vi "Heater.vi"(0 "Heater in":refnum<class "Heater_v2.lvclass">, 1 "Z_ASetState":T4, 2 "ALRs":bool[](array[boolean])=[FALSE, FALSE, FALSE], 5 "ZY_control":T3 {"Y_H" step=1.0; "SP" step=0.01 format="%.2f"}, 7 "PV":dbl step=0.01 format="%.2f", 9 "PV state":T2, 11 "error in (no error)":errorcluster, 12 "ALR_Status":T1[](array[typedef]), 13 "DI":bool[](array[boolean])) -> (4 "Heater out":refnum<class "Heater_v2.lvclass">, 6 "ZY_State":T6 {"Y"."Y_Set" format="%.2f"; "Y"."SP" step=0.01 format="%.2f"; "Y"."Y" format="%.2f"; "Y"."PV" step=0.01 format="%.2f"; "Y"."SP_Set" step=0.01 format="%.2f"}, 8 "Y":dbl format="%.2f", 10 "YB":bool[](array[boolean]), 14 "ALR_ON":bool[](array[boolean]), 15 "error out":errorcluster)   [LabVIEW 2019, in "Heater_v2.lvclass"]
uses:
  Heater_v2.lvclass
  ctl/Z_State.ctl
  Heating.lvlib
  Alarms/Ctl/ALR_Status_short.ctl
  Alarms/Alarms.lvlib
  Inputs/Ctl/Parameter State short.ctl
  Inputs/Inputs.lvlib
  ctl/Y_state.ctl
  ctl/Y_source.ctl
  ctl/Y_short.ctl
  ctl/ZM_State.ctl
  ctl/Z_source.ctl
  ctl/Z.ctl
  ctl/ZY_state_short.ctl
  REG/HE_reg.lvclass
  HE_state_v2/HE_state_v2.lvclass
  C:/my_projects/projects/Algorithms/Labview/19/Heating/heating1/HE_state_v2/HE_state_v2.lvclass
  C:/my_projects/projects/Algorithms/Labview/19/Heating/heating1/Z_state_v2/HE_Z_state_v2.lvclass
  C:/my_projects/projects/Algorithms/Labview/19/Heating/heating1/ZM_state/HE_ZM_state.lvclass
  C:/my_projects/projects/Algorithms/Labview/19/Sequence/State/State.lvclass
  ctl/ZY_control.ctl
panel:
  # "0 bit - Alarm level 1\n1 bit - Alarm level 2\n2 bit - Alarm level 3"
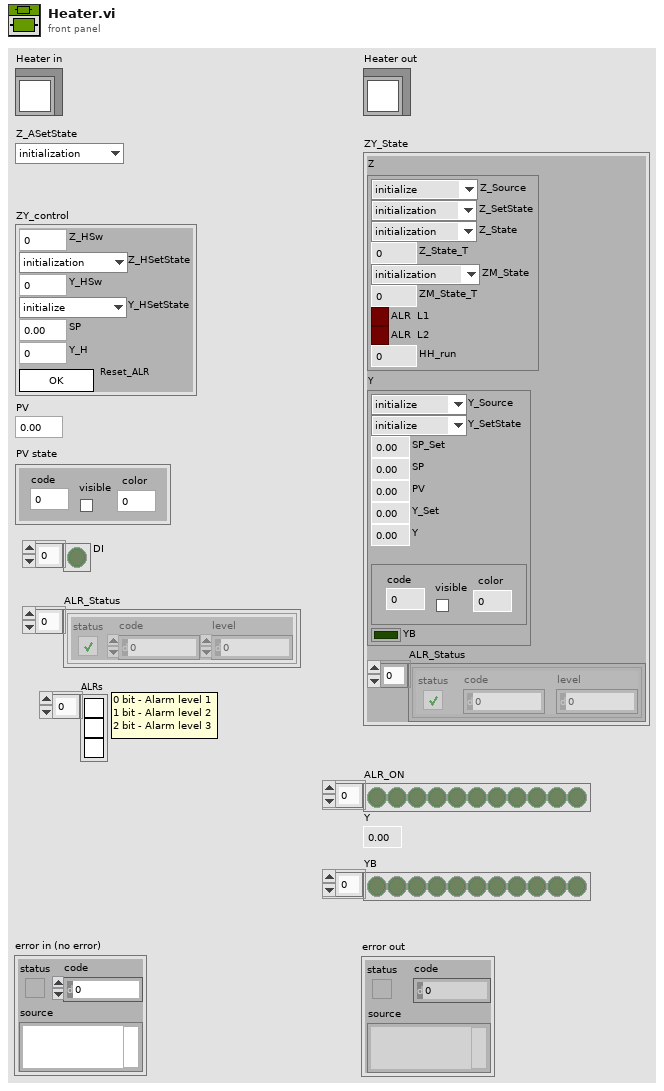
[diagram p1: front panel]
types:
  T1 = typedef "Alarms.lvlib/ALR_Status_short.ctl" = cluster{"status":bool, "code":i32, "level":i32}
  T2 = typedef "Inputs.lvlib/Parameter State short.ctl" = cluster{"code":i32, "visible":bool, "color":u32}
  T3 = typedef "Heating.lvlib/ZY_control.ctl" = cluster{"Z_HSw":u8, "Z_HSetState":T4, "Y_HSw":u8, "Y_HSetState":T5, "SP":dbl, "Y_H":dbl, "Reset_ALR":bool}
  T4 = typedef "Heating.lvlib/Z_State.ctl" = enum8{"initialization", "alarm", "disabled", "not ready", "stop ready", "reserv", "switched off", "reserv2", "switched on", "check", "on min", "decrease out", "on", "increase out", "on max"}
  T5 = typedef "Heating.lvlib/Y_state.ctl" = enum8{"initialize", "alarm", "min", "stop", "hand", "auto", "max"}
  T6 = typedef "Heating.lvlib/ZY_state_short.ctl" = cluster{"Z":T7, "Y":T10, "ALR_Status":T1[]}
  T7 = typedef "Heating.lvlib/Z.ctl" = cluster{"Z_Source":T8, "Z_SetState":T4, "Z_State":T4, "Z_State_T":u32, "ZM_State":T9, "ZM_State_T":u32, "ALR  L1":bool, "ALR  L2":bool, "HH_run":u64}
  T8 = typedef "Heating.lvlib/Z_source.ctl" = enum8{"initialize", "local disabled", "local hand", "hand", "auto", "dist"}
  T9 = typedef "Heating.lvlib/ZM_State.ctl" = enum8{"initialization", "stop", "start_cmd", "contactor_on_cmd", "heating", "on", "stop_cmd", "power_down", "contactor_off_cmd", "cooling", "restart_delay"}
  T10 = typedef "Heating.lvlib/Y_short.ctl" = cluster{"Y_Source":T11, "Y_SetState":T5, "SP_Set":dbl, "SP":dbl, "PV":dbl, "Y_Set":dbl, "Y":dbl, "Y_State":T2, "YB":bool}
  T11 = typedef "Heating.lvlib/Y_source.ctl" = enum8{"initialize", "local disabled", "local hand", "hand", "auto", "dist"}
  T12 = typedef "Heating.lvlib/Z_control.ctl" = cluster{"Z_HSw":u8, "Z_HSetState":T4, "Z_ASetState":T4, "Z_DSetState":T4}
  T13 = typedef "Heating.lvlib/Y_control.ctl" = cluster{"Y_HSw":u8, "Y_HSetState":T5, "Y_ASetState":T5, "Y_DSetState":T5}
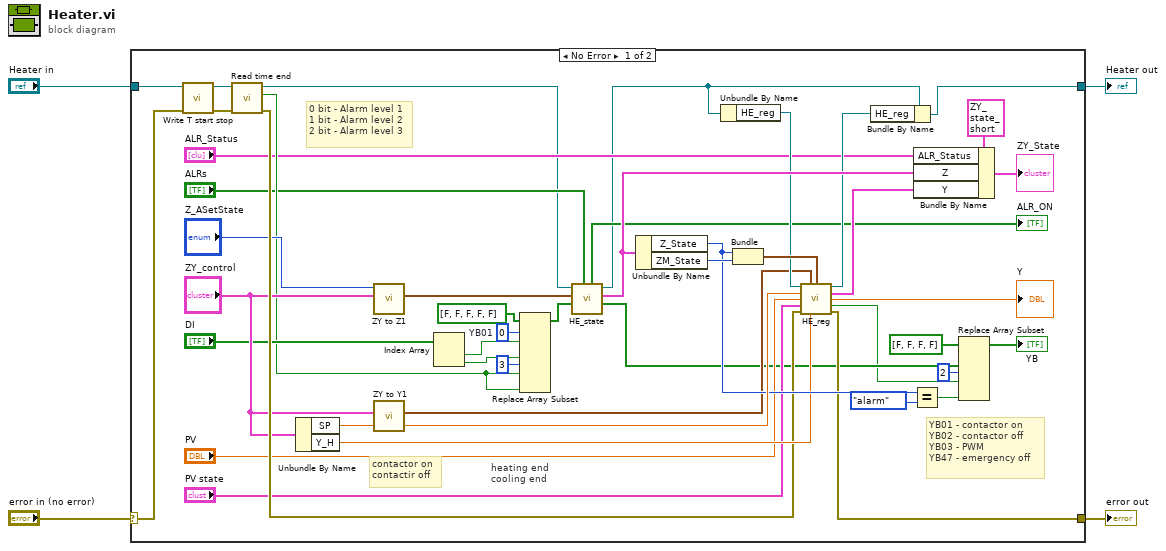
[diagram p0: block diagram]
diagram:
  n1 = case shown="No Error" "error in (no error)" {
    selector: "error in (no error)" -> [w29 w51]
    tunnel: [w27 w51] -> w3
    tunnel: [w30 w50] -> w1
    tunnel: "Heater in" -> [w25 w50]
    frame No Error {
      w49 = 0  # YB01
      # "0 bit - Alarm level 1\n1 bit - Alarm level 2\n2 bit - Alarm level 3"
      # "YB01 - contactor on\nYB02 - contactor off\nYB03 - PWM\nYB47 - emergency off"
      # "contactor on\ncontactir off"
      # "heating end\ncooling end"
      n2 = call "Write T start stop.vi"("error in (no error)"=w29, "Heater in"=w25) -> ("error out"=w33:errorcluster, "Heater out"=w34:refnum<class "Heater_v2.lvclass">)  [unwired: 8 in]
      n3 = call "Read time end.vi"("error in (no error)"=w33, "Heater in"=w34) -> ("error out"=w28:errorcluster, "End"=w10:bool, "Heater out"=w6:refnum<class "Heater_v2.lvclass">)  [unwired: 7 in]
      n4 = Unbundle By Name("ZY_control") -> ("SP"=w41:dbl, "Y_H"=w35:dbl)
      n5 = call "ZY to Z1.vi"("ZY_control"="ZY_control", "Z_ASetState"="Z_ASetState") -> ("Z_control"=w22:T12)  [unwired: 9 in]
      n6 = call "ZY to Y1.vi"("ZY_control"="ZY_control") -> ("Y"=w20:T13)  [unwired: 10 in]
      n7 = Index Array ("YB01")(array="DI") -> (element #1=w36:bool, element #2=w9:bool)  [unwired: 2 in]
      n8 = Replace Array Subset(array=bool[] [FALSE, FALSE, FALSE, FALSE, FALSE] ("XB"), new element #1=w36, index #1=w49, new element #2=w9, new element #3=w10, index #3=3 ("he end"), new element #4=w10) -> (w37:bool[])  [unwired: 2 in]
      n9 = call "HE_state.vi"("Alarm"="ALRs", "XB"=w37, "Z_control"=w22, "HE_state_in"=w6) -> ("YB"=w17:bool[], "Z"=w44:T7, "HE_state_out"=w5:refnum<class "Heater_v2.lvclass">, "ALR_ON"=→"ALR_ON":bool[])  [unwired: 4 in]
      n10 = Unbundle By Name(w44) -> ("Z_State"=w38:T4, "ZM_State"=w46:T9)
      n11 = Unbundle By Name(w5) -> ("HE_reg"=w32:refnum<class "HE_reg.lvclass">)
      n12 = Bundle("Z_State"=w38, "ZM_State"=w46) -> (w45:cluster{"Z_State":T4, "ZM_State":T9})  [unwired: 1 in]
      n13 = call "HE_reg.vi"("HE_reg in"=w32, "Y"=w20, "Z"=w45, "SP"=w41, "PV"="PV", "PV_State"="PV state", "error in (no error)"=w28, "Y_H"=w35) -> ("HE_reg out"=w31:refnum<class "HE_reg.lvclass">, "Y_State"=w43:T10, "Y"=→"Y":dbl, "YB"=w16:bool, "error out"=w27:errorcluster)  [unwired: 3 in]
      n14 = Bundle By Name(cluster=w5, "HE_reg"=w31) -> (w30:refnum<class "Heater_v2.lvclass">)
      n15 = Equal?(x=w38, y=Z_State."alarm" ("Z_State")) -> (x = y?=w13:bool)
      n16 = Bundle By Name(cluster=T6 {"Z"={"Z_Source"=enum."local disabled", "Z_SetState"=enum."on", "Z_State"=enum."alarm", "Z_State_T"=0, "ZM_State"=enum."initialization", "ZM_State_T"=0, "ALR  L1"=FALSE, "ALR  L2"=FALSE, "HH_run"=0}, "Y"={"Y_Source"=enum."local disabled", "Y_SetState"=enum."auto", "SP_Set"=0.0, "SP"=0.0, "PV"=0.0, "Y_Set"=0.0, "Y"=0.0, "Y_State"={"code"=0, "visible"=FALSE, "color"=0}, "YB"=FALSE}, "ALR_Status"=[]} ("ZY_State"), "ALR_Status"="ALR_Status", "Z"=w44, "Y"=w43) -> (→"ZY_State":T6)
      n17 = Replace Array Subset(array=bool[] [FALSE, FALSE, FALSE, FALSE], new element #1=w17, new element #2=w16, index #2=2 ("index"), new element #3=w13) -> (→"YB":bool[])  [unwired: 2 in]
    }
    frame Error {
    }
  }
  "error out" <- w3
  "Heater out" <- w1
